vi "运维调试_雷达流速仪.vi"() -> ()   [LabVIEW 2016, in "雷达流速仪.lvlib"]
uses:
  <vilib>/Utility/config.llb/NI_LVConfig.lvlib
panel:
  out "串口号":string
  in  "雷达流速仪设置":bool
  out "显示":T1
  out "通讯":bool
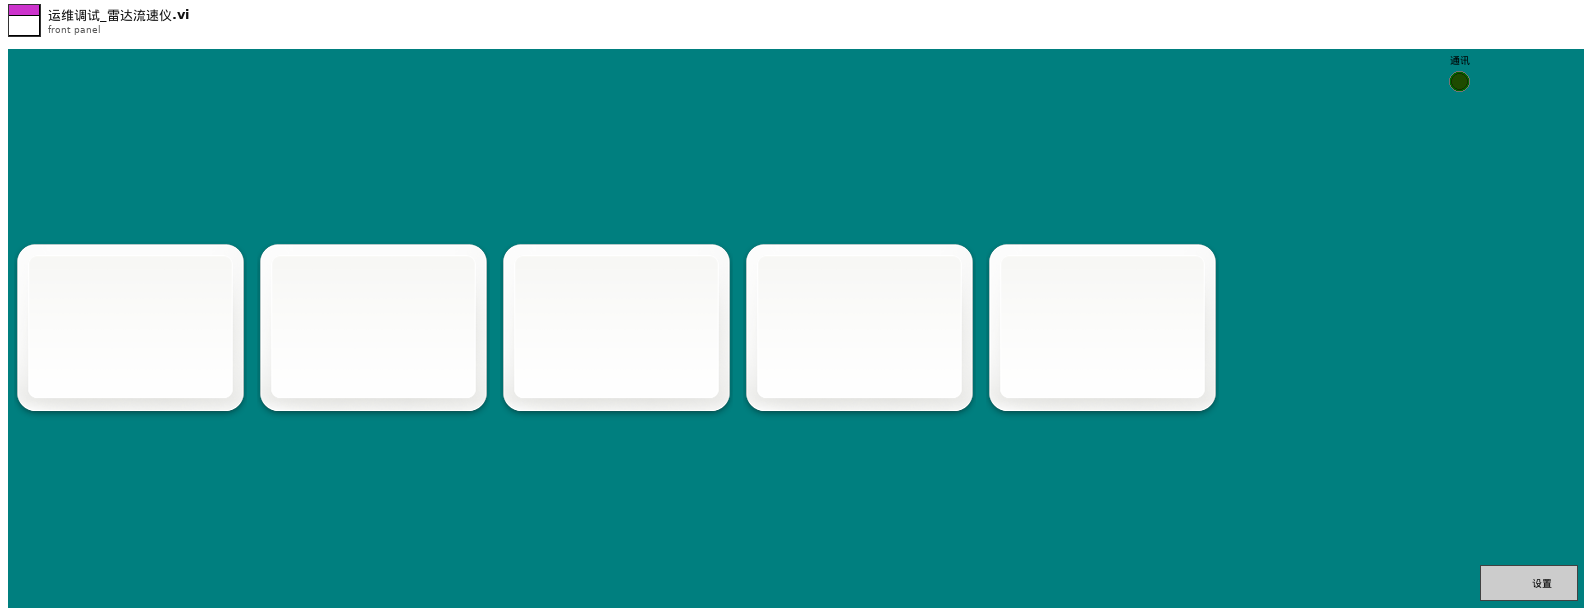
[diagram p1: front panel]
types:
  T1 = typedef "多数值显示.ctl" = cluster{"显示":T2, "显示 2":T2, "显示 3":T2, "显示 4":T2, "显示 5":T2, "显示 6":T2, "显示 12":T2, "显示 11":T2, "显示 10":T2, "显示 9":T2, "显示 8":T2, "显示 7":T2}
  T2 = typedef "数值显示.ctl" = cluster{"中文项目名称":string, "英文项目名称":string, "浓度":string, "单位":string}
  T3 = typedef "NI_LVConfig.lvlib/Config Data RefNum.ctl" = refnum<k1>
  T4 = cluster{"时间":timestamp, "水位":dbl, "流速":dbl, "瞬时流量":dbl, "正累积流量":dbl, "负累积流量":dbl}
  T5 = typedef "LVDateTimeRec.ctl" = cluster{"秒数的小数部分":dbl, "秒":i32, "分":i32, "时":i32, "日":i32, "月":i32, "年":i32, "天数（周）":i32, "天数（年）":i32, "DST":i32}
  T6 = cluster{"采集数据[0]":sgl, "采集数据[1]":sgl, "采集数据[2]":sgl, "采集数据[3]":sgl, "采集数据[4]":sgl}
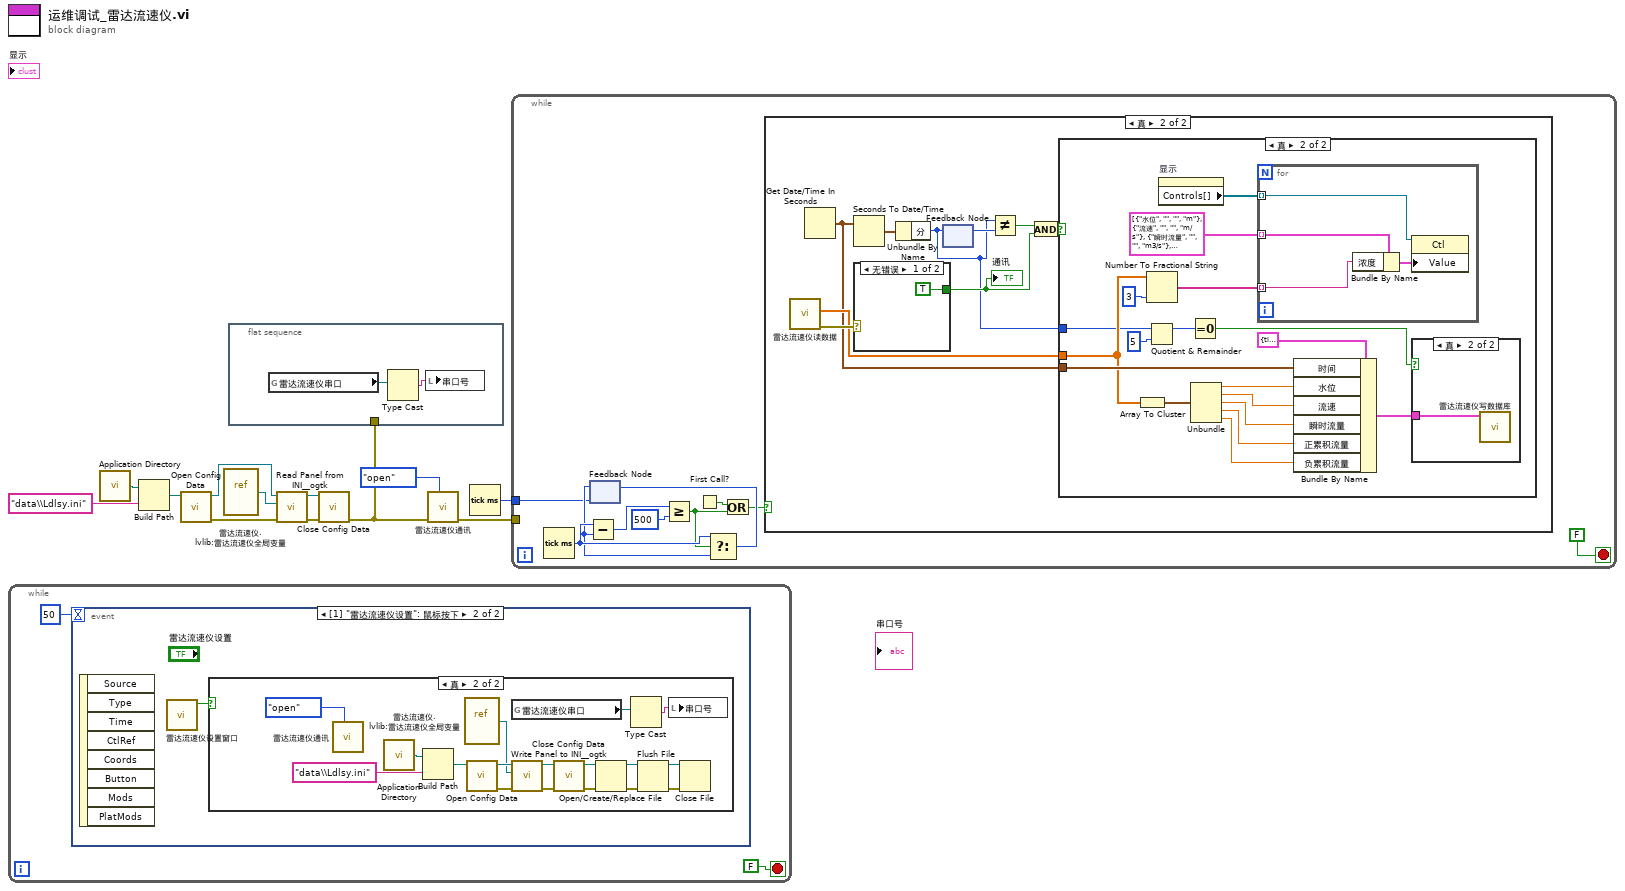
[diagram p0: block diagram]
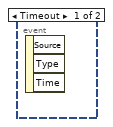
[diagram p2: hidden frame]
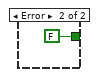
[diagram p7: hidden frame]
diagram:
  n1 = while {
    stop <- FALSE stop-if-true
    n2 = event shown="[1] \"雷达流速仪设置\": 鼠标按下" {
      selector: _ -> [_ _]
      dyn-events: _ -> [_ _]
      timeout: 50 -> [_ _]
      event Timeout {
        n3 = event-data() -> ()  [unwired: 1 in, 3 out]
      }
      event "雷达流速仪设置": Mouse Down {
        n4 = event-data() -> ()  [unwired: 1 in, 8 out]
        n5 = call "雷达流速仪设置窗口.vi"() -> ("确定输出"=w15:bool)  [unwired: 11 in]
        n6 = case shown="真" w15 {
          frame False {
          }
          frame True {
            n7 = call "雷达流速仪通讯.vi"("STEP"=enum16{"open", "read", "write", "close"}."open") -> ()  [unwired: 8 in, 3 out]
            n8 = call <vilib>:"Application Directory.vi"() -> ("Application Directory"=w31:path)
            n9 = Build Path(base path=w31, name or relative path="data\\Ldlsy.ini" ("名称或相对路径")) -> (appended path=w29:path)
            n10 = vi-ref "雷达流速仪.lvlib:雷达流速仪全局变量.vi"() -> (w18:refnum<vi>)
            n11 = call <vilib>:"Open Config Data.vi"("configuration file path"=w29) -> ("error out"=w19:errorcluster, "refnum"=w20:T3)  [unwired: 8 in, 1 out]
            n12 = global read "雷达流速仪全局变量.vi" "雷达流速仪串口"() -> (w17:refnum<visa-resource-name>)
            n13 = call <userlib>:"Write Panel to INI__ogtk.vi"("error in (no error)"=w19, "VI ref"=w18, "refnum"=w20) -> ("error out"=w22:errorcluster, "refnum out"=w21:T3)  [unwired: 7 in]
            n14 = call <vilib>:"Close Config Data.vi"("error in (no error)"=w22, "refnum"=w21) -> ("error out"=w27:errorcluster, "file path"=w28:path)  [unwired: 8 in]
            n15 = Open/Create/Replace File(file path (use dialog)=w28, error in=w27) -> (refnum out=w24:refnum<file>, error out=w23:errorcluster)  [unwired: 4 in, 1 out]
            n16 = Type Cast(x=w17) -> (*(type *) &x=w16:string)  [unwired: 1 in]
            n17 = Flush File(refnum=w24, error in=w23) -> (refnum out=w25:refnum<file>, error out=w26:errorcluster)
            n18 = local write "串口号"(w16) -> ()
            n19 = Close File(refnum=w25, error in=w26) -> ()  [unwired: 2 out]
          }
        }
      }
    }
  }
  n20 = call <vilib>:"Application Directory.vi"() -> ("Application Directory"=w8:path)
  n21 = Build Path(base path=w8, name or relative path="data\\Ldlsy.ini" ("名称或相对路径")) -> (appended path=w10:path)
  n22 = call <vilib>:"Open Config Data.vi"("configuration file path"=w10) -> ("error out"=w6:errorcluster, "refnum"=w11:T3)  [unwired: 8 in, 1 out]
  n23 = vi-ref "雷达流速仪.lvlib:雷达流速仪全局变量.vi"() -> (w5:refnum<vi>)
  n24 = flat-sequence {
    tunnel: w1 -> [_]
    frame #0 {
      n25 = global read "雷达流速仪全局变量.vi" "雷达流速仪串口"() -> (w33:refnum<visa-resource-name>)
      n26 = Type Cast(x=w33) -> (*(type *) &x=w34:string)  [unwired: 1 in]
      n27 = local write "串口号"(w34) -> ()
    }
  }
  n28 = call <userlib>:"Read Panel from INI__ogtk.vi"("error in (no error)"=w6, "VI ref"=w5, "refnum"=w11) -> ("error out"=w7:errorcluster, "refnum out"=w12:T3)  [unwired: 7 in]
  n29 = call <vilib>:"Close Config Data.vi"("error in (no error)"=w7, "refnum"=w12) -> ("error out"=w1:errorcluster)  [unwired: 8 in, 1 out]
  n30 = call "雷达流速仪通讯.vi"("STEP"=enum16{"open", "read", "write", "close"}."open", "Error in"=w1) -> ("error out"=w3:errorcluster)  [unwired: 7 in, 2 out]
  n31 = Tick Count (ms)() -> (millisecond timer value=w2:u32)
  n32 = while {
    tunnel: w3 -> [_]
    tunnel: w2 -> [w37]
    stop <- FALSE stop-if-true
    n33 = Tick Count (ms)() -> (millisecond timer value=w42:u32)
    n34 = feedback #1(w37) -> (w41:u32)
    n35 = Subtract(x=w42, y=w41) -> (x-y=w44:u32)
    n36 = Greater Or Equal?(x=w44, y=u32 500) -> (x >= y?=w38:bool)
    n37 = First Call?() -> (First Call?: T/F=w39:bool)
    n38 = Select(t=w42, s=w38, f=w41) -> (s? t:f=w40:u32)
    n39 = feedback-in #1(w40) -> ()
    n40 = Or(x=w39, y=w38) -> (x .or. y?=w36:bool)
    n41 = case shown="真" w36 {
      frame False {
      }
      frame True {
        n42 = call "雷达流速仪读数据.vi"() -> ("error out"=w48:errorcluster, "采集数据"=w47:sgl[])  [unwired: 8 in]
        n43 = Get Date/Time In Seconds() -> (seconds since 1Jan1904=w46:timestamp)
        n44 = Seconds To Date/Time(time stamp (now)=w46) -> (date time rec=w52:T5)  [unwired: 1 in]
        n45 = case shown="无错误" w48 {
          tunnel: [TRUE FALSE] -> w50
          frame No Error {
          }
          frame Error {
          }
        }
        "通讯" <- w50
        n46 = Unbundle By Name(w52) -> ("分"=w45:i32)
        n47 = feedback #2() -> (w53:i32)  [unwired: 1 in]
        n48 = feedback-in #2(w45) -> ()
        n49 = Not Equal?(x=w45, y=w53) -> (x != y?=w51:bool)
        n50 = And(x=w51, y=w50) -> (x .and. y?=w49:bool)
        n51 = case shown="真" w49 {
          tunnel: w47 -> [_ w66]
          tunnel: w46 -> [_ w69]
          tunnel: w45 -> [_ w58]
          frame False {
          }
          frame True {
            n52 = Array To Cluster(array=w66) -> (cluster=w65:T6)
            n53 = Number To Fractional String(number=w66, precision (6)=i16 3 ("精度(6)")) -> (F-format string=w67:string[])  [unwired: 2 in]
            n54 = Quotient & Remainder(x=w58, y=5) -> (x-y*floor(x/y)=w56:i32)  [unwired: 1 out]
            n55 = property on="显示" class="Clust (严格)"() -> ("Controls[]"=w68:refnum<vi>[])  [unwired: 2 in, 2 out]
            n56 = Equal To 0?(x=w56) -> (x = 0?=w55:bool)
            n57 = Unbundle(w65) -> ("采集数据[0]"=w64:sgl, "采集数据[1]"=w63:sgl, "采集数据[2]"=w62:sgl, "采集数据[3]"=w61:sgl, "采集数据[4]"=w60:sgl)
            n58 = for {
              tunnel: w68 -> [w75] mode=indexing
              tunnel: T2[] [{"中文项目名称"="水位", "英文项目名称"="", "浓度"="", "单位"="m"}, {"中文项目名称"="流速", "英文项目名称"="", "浓度"="", "单位"="m/s"}, {"中文项目名称"="瞬时流量", "英文项目名称"="", "浓度"="", "单位"="m3/s"}, {"中文项目名称"="正累积流量", "英文项目名称"="", "浓度"="", "单位"="m3"}, {"中文项目名称"="负累积流量", "英文项目名称"="", "浓度"="", "单位"="M3"}] -> [w76] mode=indexing
              tunnel: w67 -> [w73] mode=indexing
              n59 = Bundle By Name(cluster=w76, "浓度"=w73) -> (w74:T2)
              n60 = property class="Ctl"(reference=w75, "Value"=w74) -> ()  [unwired: 1 in, 2 out]
            }
            n61 = Bundle By Name(cluster=T4 {"时间"=timestamp(3777000960.083023 s since 1904-01-01), "水位"=0.0, "流速"=0.0, "瞬时流量"=0.0, "正累积流量"=0.0, "负累积流量"=0.0} ("输出簇"), "时间"=w69, "水位"=w64, "流速"=w63, "瞬时流量"=w62, "正累积流量"=w61, "负累积流量"=w60) -> (w59:T4)
            n62 = case shown="真" w55 {
              tunnel: w59 -> [_ w72]
              frame False {
              }
              frame True {
                n63 = call "雷达流速仪写数据库.vi"("采集数据"=w72) -> ()  [unwired: 10 in, 1 out]
              }
            }
          }
        }
      }
    }
  }
